vi "niFPGA Quantizer.vi"(2 "input":i32) -> (7 "output":i32)   [LabVIEW 2017]
doc: "Quantizes an integer input signal using fixed-point rounding."
uses:
  <vilib>/express/rvi/analysis/control/nonlinear/nirviQuantizationModes.ctl
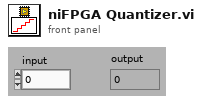
[diagram p1: front panel]
types:
  T1 = typedef "nirviQuantizationModes.ctl" = enum32{"Round to nearest", "One bit round", "Truncate", "No rounding"}
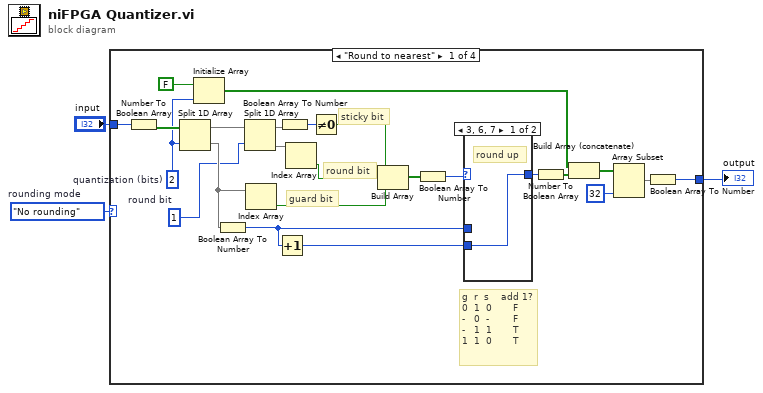
[diagram p0: block diagram]
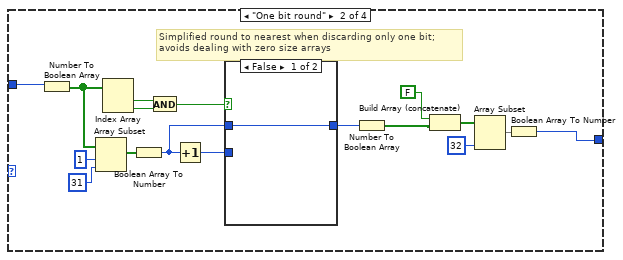
[diagram p3: hidden frame]
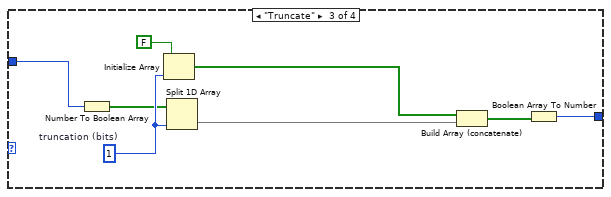
[diagram p5: hidden frame]
diagram:
  w1 = nirviQuantizationModes."No rounding"  # rounding mode
  n1 = case shown="\"Round to nearest\"" w1 {
    tunnel: "input" -> [w27 w46 w51 w57]
    tunnel: [w26 w30 w50 w57] -> w2
    frame "Round to nearest" {
      w4 = 1  # round bit
      w5 = i8 2  # quantization (bits)
      # "g  r  s    add 1?\n0  1  0       F\n-   0  -        F\n-   1  1       T\n1  1  0       T"
      # "guard bit"
      # "round bit"
      # "sticky bit"
      n2 = Number To Boolean Array(number=w27) -> (Boolean array=w25:bool[])
      n3 = Split 1D Array(array=w25, index=w5) -> (first subarray=w24:bool[], second subarray=w20:bool[])
      n4 = Initialize Array(FALSE, w5) -> (w9:bool[])
      n5 = Boolean Array To Number(Boolean array=w20) -> (number=w12:u32)
      n6 = Split 1D Array(array=w24, index=w4) -> (first subarray=w23:bool[], second subarray=w21:bool[])
      n7 = Index Array(array=w20) -> (element=w17:bool)  [unwired: 1 in]
      n8 = Increment(x=w12) -> (x+1=w13:u32)
      n9 = Boolean Array To Number(Boolean array=w23) -> (number=w22:u8)
      n10 = Index Array(array=w21) -> (element=w18:bool)  [unwired: 1 in]
      n11 = Not Equal To 0?(x=w22) -> (x != 0?=w19:bool)
      n12 = Build Array(w19, w18, w17) -> (w16:bool[])
      n13 = Boolean Array To Number(Boolean array=w16) -> (number=w15:u8)
      n14 = case shown="3, 6, 7" w15 {
        tunnel: [w28 w29] -> w14
        tunnel: w12 -> [_ w29]
        tunnel: w13 -> [w28 _]
        frame 3, 6, 7 {
          # "round up"
        }
        frame Default {
        }
      }
      n15 = Number To Boolean Array(number=w14) -> (Boolean array=w11:bool[])
      n16 = Build Array (concatenate)(w9, w11) -> (w7:bool[])
      n17 = Array Subset(array=w7, length=32) -> (w8:bool[])  [unwired: 1 in]
      n18 = Boolean Array To Number(Boolean array=w8) -> (number=w26:u32)
    }
    frame "One bit round" {
      # "Simplified round to nearest when discarding only one bit;\navoids dealing with zero size arrays"
      n19 = Number To Boolean Array(number=w46) -> (Boolean array=w43:bool[])
      n20 = Array Subset(array=w43, index=1, length=31) -> (w40:bool[])
      n21 = Index Array(array=w43) -> (element #1=w44:bool, element #2=w45:bool)  [unwired: 2 in]
      n22 = Boolean Array To Number(Boolean array=w40) -> (number=w37:u32)
      n23 = And(x=w44, y=w45) -> (x .and. y?=w39:bool)
      n24 = Increment(x=w37) -> (x+1=w38:u32)
      n25 = case shown="False" w39 {
        tunnel: w38 -> [_ w48]
        tunnel: w37 -> [w47 _]
        tunnel: [w47 w48] -> w32
        frame False {
        }
        frame True {
        }
      }
      n26 = Number To Boolean Array(number=w32) -> (Boolean array=w36:bool[])
      n27 = Build Array (concatenate)(FALSE, w36) -> (w34:bool[])
      n28 = Array Subset(array=w34, length=32) -> (w35:bool[])  [unwired: 1 in]
      n29 = Boolean Array To Number(Boolean array=w35) -> (number=w30:u32)
    }
    frame "Truncate" {
      w55 = i8 1  # truncation (bits)
      n30 = Number To Boolean Array(number=w51) -> (Boolean array=w54:bool[])
      n31 = Initialize Array(FALSE, w55) -> (w53:bool[])
      n32 = Split 1D Array(array=w54, index=w55) -> (second subarray=w56:bool[])  [unwired: 1 out]
      n33 = Build Array (concatenate)(w53, w56) -> (w49:bool[])
      n34 = Boolean Array To Number(Boolean array=w49) -> (number=w50:u32)
    }
    frame "No rounding", Default {
    }
  }
  "output" <- w2
